vi "RT Loop - Watchdog.vi"(11 "Message Queue":refnum<queue> caption="消息队列") -> ()   [LabVIEW 2013]
uses:
  support/Message Queue/Message Cluster.ctl
  <vilib>/RTwatchdog.llb/Watchdog expiration actions.ctl
  <vilib>/RTwatchdog.llb/Watchdog status enum.ctl
  Globals/Global - Configuration Options.vi
  Globals/Global - All RT Loop Stop.vi
  support/Message Queue/Message Queue.lvlib
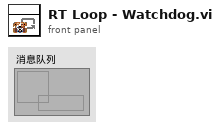
[diagram p1: front panel]
types:
  T1 = typedef "Watchdog status enum.ctl" = enum16{"disabled", "expired", "running"}
  T2 = typedef "Watchdog expiration actions.ctl" = cluster{"reset":bool, "occurrence":bool, "trigger protocol":enum16{"active high", "active low", "open collector"}, "trigger line":enum16{"none", "line 0", "line 1", "line 2", "line 3", "line 4", "line 5", "line 6", "line 7", "SMB line 0"}, "disable watchdog on VI exit":bool}
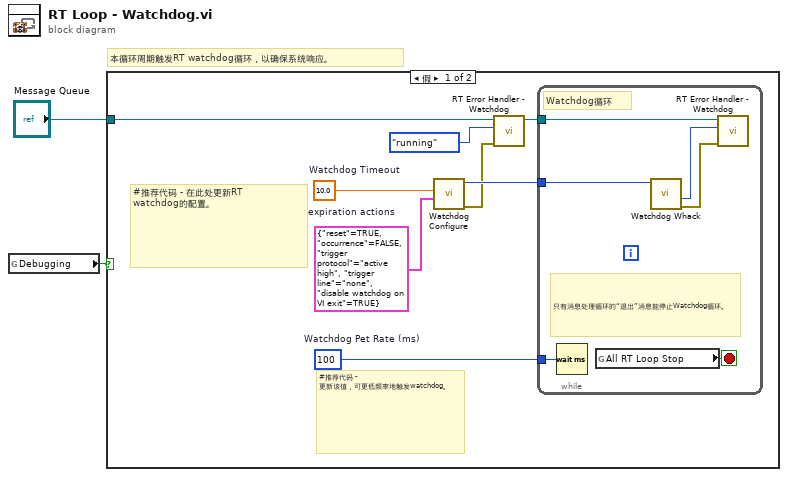
[diagram p0: block diagram]
diagram:
  # "本循环周期触发RT watchdog循环，以确保系统响应。"
  n1 = global read "Global - Configuration Options.vi" "Debugging"() -> (w1:bool)
  n2 = case shown="假" w1 {
    tunnel: "Message Queue" -> [w10 _]
    frame False {
      w4 = u32 100  # Watchdog Pet Rate (ms)
      w5 = T2 {"reset"=TRUE, "occurrence"=FALSE, "trigger protocol"=enum."active high", "trigger line"=enum."none", "disable watchdog on VI exit"=TRUE}  # expiration actions
      w6 = 10.0  # Watchdog Timeout
      # "#推荐代码 - 在此处更新RT watchdog的配置。"
      # "#推荐代码 - 更新该值，可更低频率地触发watchdog。"
      n3 = call <vilib>:"Watchdog Configure.vi"("expiration actions"=w5, "timeout (1 sec)"=w6) -> ("error out"=w7:errorcluster, "watchdogID"=w8:u32)  [unwired: 2 in, 2 out]
      n4 = call "RT Error Handler - Watchdog.vi"("error in (no error)"=w7, "watchdog status"=Watchdog_status_enum."running", "Message Queue"=w10) -> ("dup Message Queue"=w9:refnum<queue>)  [unwired: 8 in]
      n5 = while {
        tunnel: w9 -> [w15]
        tunnel: w8 -> [w13]
        tunnel: w4 -> [w14]
        stop <- w16 stop-if-true
        # "只有消息处理循环的“退出”消息能停止Watchdog循环。"
        # "Watchdog循环"
        n6 = Wait (ms)(milliseconds to wait=w14) -> ()  [unwired: 1 out]
        n7 = global read "Global - All RT Loop Stop.vi" "All RT Loop Stop"() -> (w16:bool)
        n8 = call <vilib>:"Watchdog Whack.vi"("watchdogID in"=w13) -> ("error out"=w12:errorcluster, "watchdog status"=w11:T1)  [unwired: 4 in, 1 out]
        n9 = call "RT Error Handler - Watchdog.vi"("error in (no error)"=w12, "watchdog status"=w11, "Message Queue"=w15) -> ()  [unwired: 8 in, 1 out]
      }
    }
    frame True {
      # "调试时不能启用watchdog。"
    }
  }
